vi "Add Panel Info In Reply Info.vi"(8 "error in (no error)":errorcluster, 10 "Reply":refnum<class "Console Reply.lvclass">, 11 "Console in":refnum<class "Console.lvclass">) -> (0 "error out":errorcluster, 2 "Console2API Q out":refnum<class "Console Reply.lvclass">, 3 "Console out":refnum<class "Console.lvclass">)   [LabVIEW 2015, in "EditPanel API.lvlib" / "Console.lvclass"]
uses:
  Console.lvclass
  Console Reply/Console Reply/Console Reply.lvclass
  Console.lvclass/Console.ctl
  Console Reply/Console Reply/Console Reply.lvclass/Console Reply.ctl
  <vilib>/ActorFramework/Message Enqueuer/Message Enqueuer.lvclass
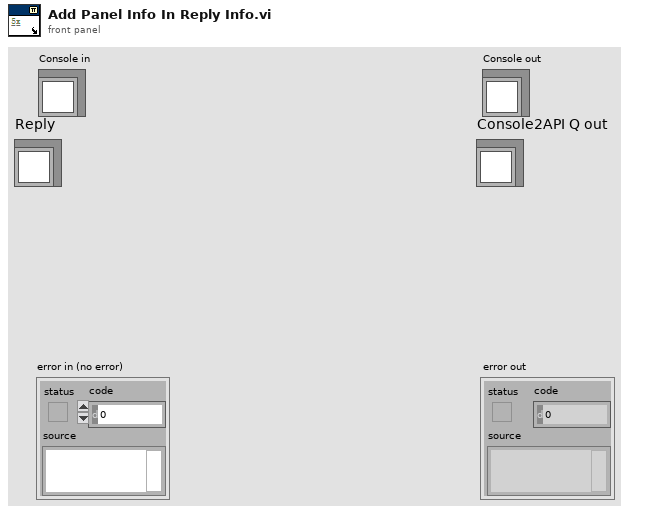
[diagram p1: front panel]
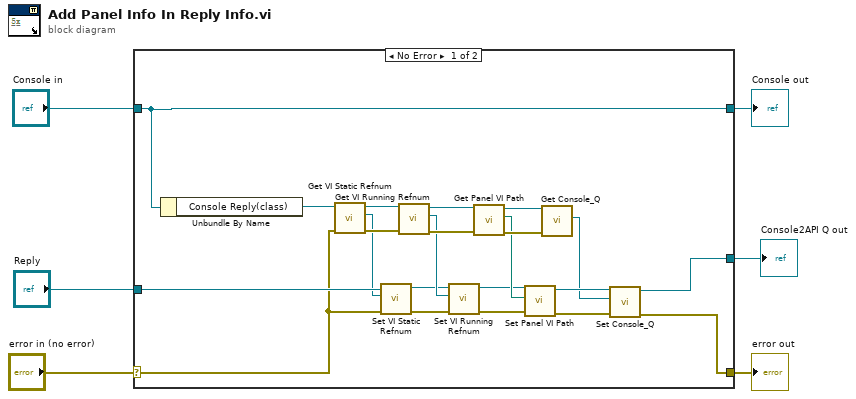
[diagram p0: block diagram]
diagram:
  n1 = case shown="No Error" "error in (no error)" {
    selector: "error in (no error)" -> [w15 w31]
    tunnel: [w7 w31] -> w5
    tunnel: [w28 w30] -> w3
    tunnel: "Console in" -> [w28 w30]
    tunnel: "Reply" -> [w22 w29]
    tunnel: [w8 w29] -> w1
    frame No Error {
      n2 = Unbundle By Name(w28) -> ("Console Reply(class)"=w27:refnum<class "Console Reply.lvclass">)
      n3 = call "Get VI Static Refnum.vi"("error in (no error)"=w15, "Console Reply in"=w27) -> ("error out"=w21:errorcluster, "VI Static Refnum"=w20:refnum<vi>, "Console Reply out"=w19:refnum<class "Console Reply.lvclass">)  [unwired: 7 in]
      n4 = call "Set VI Static Refnum.vi"("error in (no error)"=w15, "VI Static Refnum"=w20, "Console Reply in"=w22) -> ("error out"=w16:errorcluster, "Console Reply out"=w17:refnum<class "Console Reply.lvclass">)  [unwired: 7 in]
      n5 = call "Get VI Running Refnum.vi"("error in (no error)"=w21, "Console Reply.lvclass"=w19) -> ("error out"=w24:errorcluster, "VI Running Refnum"=w18:refnum<vi>, "Console Reply.lvclass out"=w26:refnum<class "Console Reply.lvclass">)  [unwired: 7 in]
      n6 = call "Set VI Running Refnum.vi"("error in (no error)"=w16, "VI Running Refnum"=w18, "Console Reply.lvclass"=w17) -> ("error out"=w12:errorcluster, "Console Reply.lvclass out"=w13:refnum<class "Console Reply.lvclass">)  [unwired: 7 in]
      n7 = call "Get Panel VI Path.vi"("error in (no error)"=w24, "Console Reply.lvclass"=w26) -> ("error out"=w23:errorcluster, "Panel VI Path"=w14:path, "Console Reply.lvclass out"=w25:refnum<class "Console Reply.lvclass">)  [unwired: 7 in]
      n8 = call "Set Panel VI Path.vi"("error in (no error)"=w12, "Panel VI Path"=w14, "Console Reply.lvclass"=w13) -> ("error out"=w10:errorcluster, "Console Reply.lvclass out"=w11:refnum<class "Console Reply.lvclass">)  [unwired: 7 in]
      n9 = call "Get Console_Q.vi"("error in (no error)"=w23, "Console Reply.lvclass"=w25) -> ("Console Q"=w9:refnum<class "Message Enqueuer.lvclass">)  [unwired: 7 in, 2 out]
      n10 = call "Set Console_Q.vi"("error in (no error)"=w10, "Console Q"=w9, "Console Reply.lvclass"=w11) -> ("error out"=w7:errorcluster, "Console Reply.lvclass out"=w8:refnum<class "Console Reply.lvclass">)  [unwired: 7 in]
    }
    frame Error {
    }
  }
  "error out" <- w5
  "Console out" <- w3
  "Console2API Q out" <- w1
